vi "Create.vi"(8 "error in (no error)":errorcluster, 10 "session":refnum<k35>) -> (0 "error out":errorcluster, 3 "Coin Analyser out":refnum<class "Coin Analyser.lvclass">)   [LabVIEW 2022 SP3, in "Coin Analyser.lvclass"]
uses:
  Coin Analyser.lvclass
  Coin Analyser.lvclass/Coin Analyser.ctl
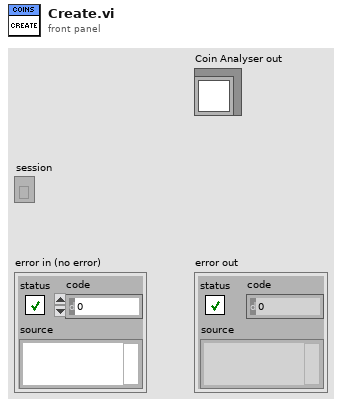
[diagram p1: front panel]
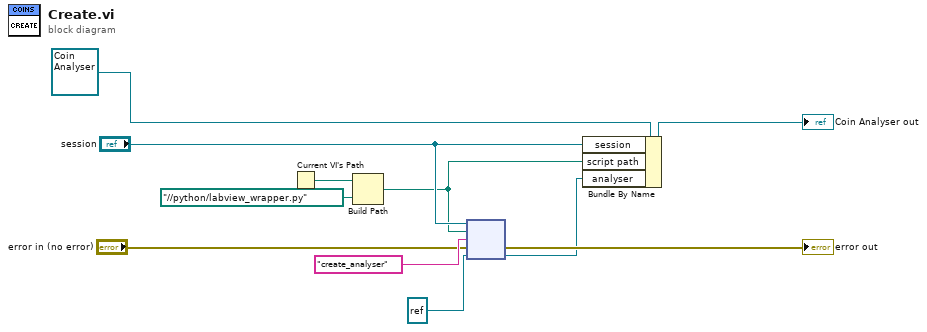
[diagram p0: block diagram]
diagram:
  n1 = Current VI's Path() -> (path=w3:path)
  n2 = Build Path(base path=w3, name or relative path=path "../../python/labview_wrapper.py") -> (appended path=w1:path)
  n3 = node("session", w1, "create_analyser" ("function name"), "error in (no error)", refnum<k38> refnum ("Python Object Refnum")) -> (→"error out":errorcluster, w4:refnum<k38>)  [unwired: 3 out]
  n4 = Bundle By Name(cluster=refnum<class "Coin Analyser.lvclass"> refnum ("Coin Analyser in"), "session"="session", "script path"=w1, "analyser"=w4) -> (→"Coin Analyser out":refnum<class "Coin Analyser.lvclass">)
